vi "close2D.vi"(8 "error in (no error)":errorcluster, 11 "xml":refnum<class "NativeXML.lvclass">[][](array[class])) -> (0 "error out":errorcluster)   [LabVIEW 2009, in "Tools.lvlib" / "xml.lvlib" / "NativeXML.lvclass"]
uses:
  NativeXML.lvclass
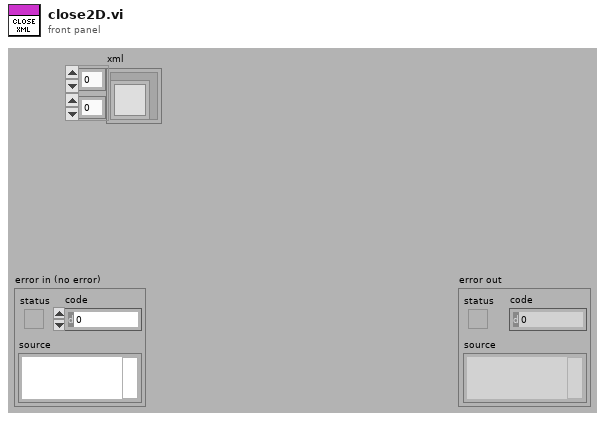
[diagram p1: front panel]
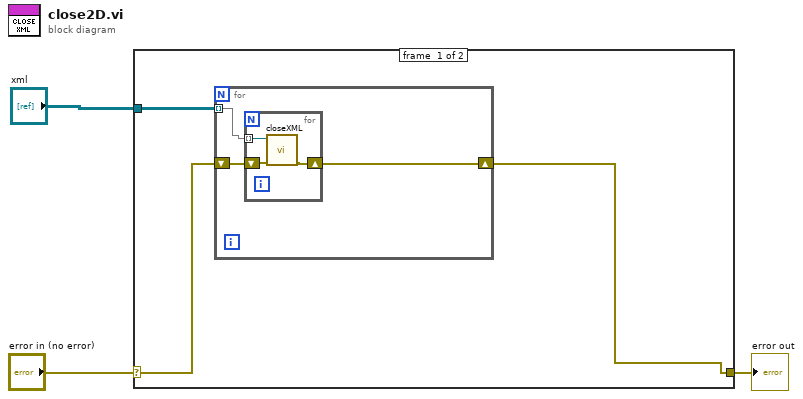
[diagram p0: block diagram]
diagram:
  n1 = case shown="No Error" "error in (no error)" {
    selector: "error in (no error)" -> [w5 w13]
    tunnel: [w4 w13] -> w2
    tunnel: "xml" -> [w6 _]
    frame #0 {
      n2 = for {
        tunnel: w6 -> [w9] mode=indexing
        shift-right: [w8] -> w4
        shift-left: w5 -> [w7]
        n3 = for {
          tunnel: w9 -> [w12] mode=indexing
          shift-right: [w11] -> w8
          shift-left: w7 -> [w10]
          n4 = call "closeXML.vi"("error in (no error)"=w10, "NativeXML in"=w12) -> ("error out"=w11:errorcluster)  [unwired: 9 in]
        }
      }
    }
    frame #1 {
    }
  }
  "error out" <- w2
